vi "ActionVIOnLoad.vi"(8 "error in (no error)":errorcluster, 11 "Device Item Ref in":T1 format="%.0x") -> (0 "error out":errorcluster, 3 "Device Item Ref out":T1 format="%.0x")   [LabVIEW 2015, in "Fuel Injector Analysis Addon System Explorer.lvlib"]
uses:
  Fuel Injector Analysis Addon System Explorer.lvlib
  <vilib>/NI Veristand/Custom Device API/Custom Device Item Ref.ctl
  NationalInstruments.VeriStand.SystemDefinitionAPI
  Shared/Constants.vi
  <vilib>/NI Veristand/Custom Device Tools/Custom Device Utility Library/NI VeriStand - Search for Item by GUID.vi
  <vilib>/NI Veristand/Custom Device Tools/Custom Device Utility Library/NI VeriStand - Search for All Items by GUID.vi
  <vilib>/NI Veristand/Custom Device API/Custom Device API.lvlib
  <vilib>/NI Veristand/Custom Device Tools/Custom Device Utility Library/Custom Device Utility Library.lvlib
  Shared/Fuel Injector Analysis Addon Shared.lvlib
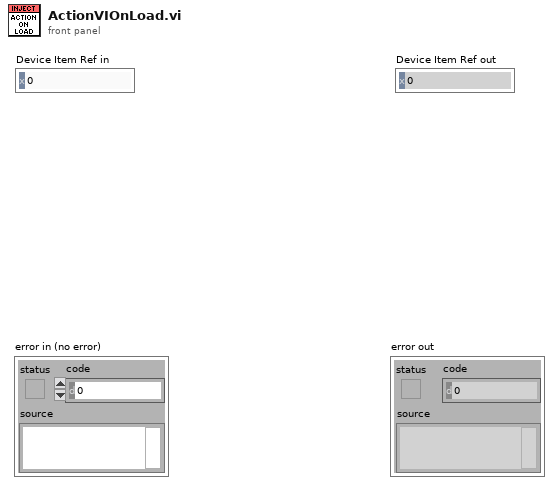
[diagram p1: front panel]
types:
  T1 = typedef "Custom Device API.lvlib/Custom Device Item Ref.ctl" = u64
  T2 = typedef "Fuel Injector Analysis Addon Shared.lvlib/Analysis.Channels.Select.ctl" = cluster{"Pull In Time":bool, "Pull In Max Current":bool, "Pull In Max Voltage":bool, "Pull In Min Voltage":bool, "Pull In Avg Voltage":bool, "Hold Time":bool, "Hold Max Current":bool, "Hold Min Current":bool, "Hold Avg Current":bool, "Hold Max Voltage":bool, "Hold Min Voltage":bool, "Hold Avg Max Voltage":bool, "Hold Avg Min Voltage":bool, "Off Time":bool, "Off Max Current":bool, "Off Min Current":bool, "Off Avg Current":bool, "Off Max Voltage":bool, "Off Min Voltage":bool, "Off Avg Voltage":bool, "Total Voltage Pulses":bool, "Total Stage Time":bool}
  T3 = typedef "Custom Device API.lvlib/Custom Device Item Info.ctl" = cluster{"Name":string, "Is Channel":bool, "GUID":string, "Is Waveform":bool}
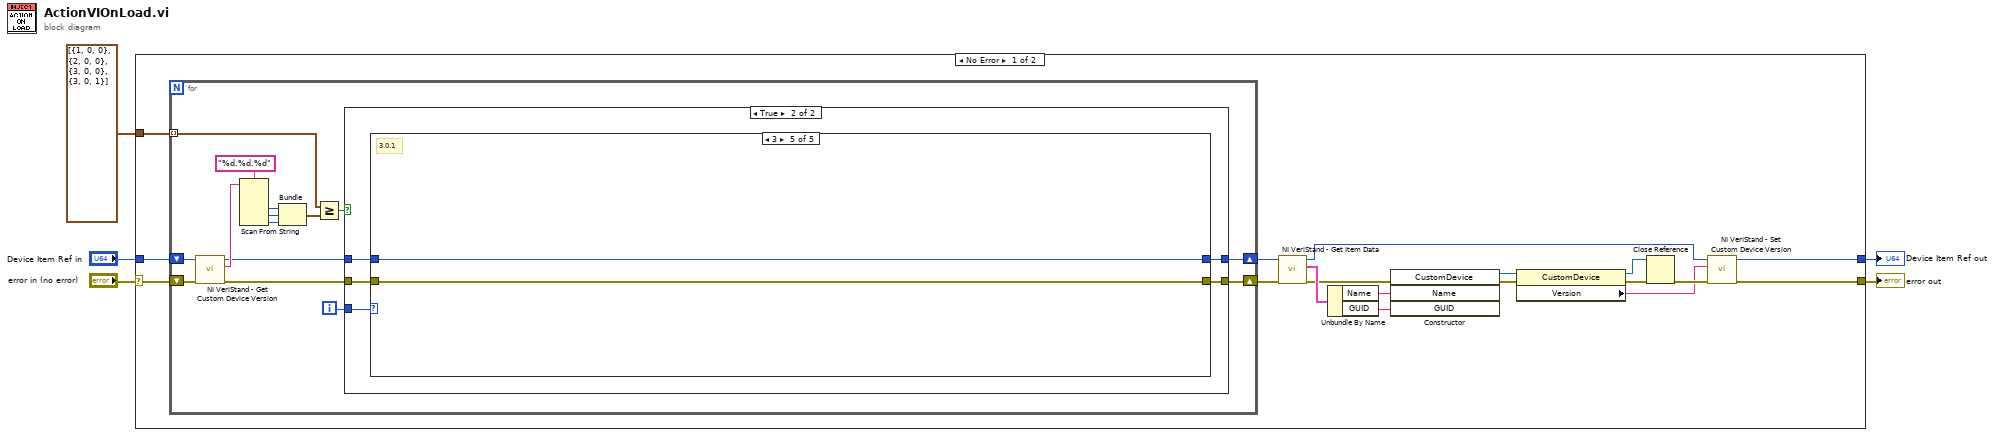
[diagram p0: block diagram]
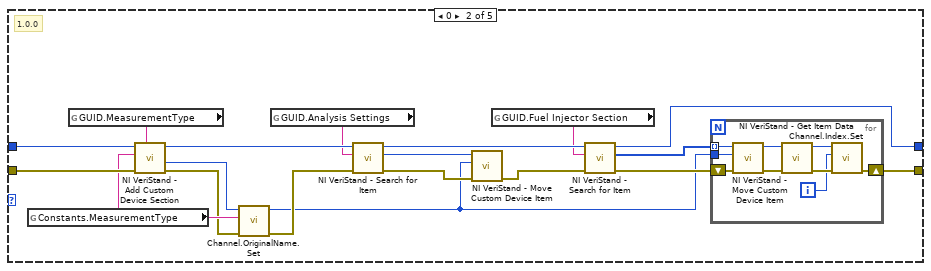
[diagram p4: hidden frame]
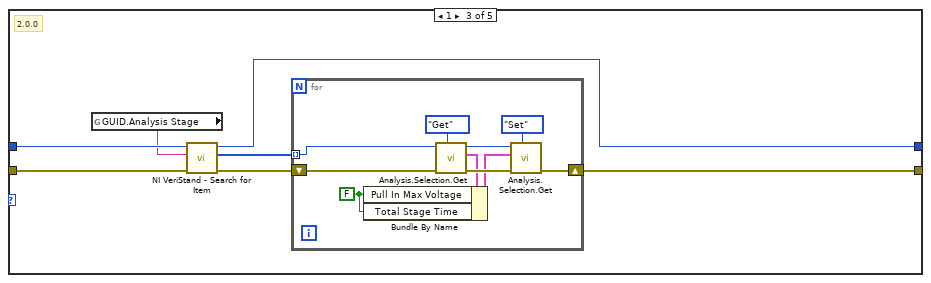
[diagram p5: hidden frame]
diagram:
  n1 = case shown="No Error" "error in (no error)" {
    selector: "error in (no error)" -> [w22 w98]
    tunnel: [w8 w98] -> w2
    tunnel: "Device Item Ref in" -> [w21 w97]
    tunnel: [w6 w97] -> w1
    tunnel: cluster{i32, i32, i32}[] [{1, 0, 0}, {2, 0, 0}, {3, 0, 0}, {3, 0, 1}] -> [w23 _]
    frame No Error {
      n2 = for {
        tunnel: w23 -> [w26] mode=indexing
        shift-right: [w31] -> w9
        shift-left: w22 -> [w36]
        shift-right: [w29] -> w7
        shift-left: w21 -> [w35]
        i -> [w28]
        n3 = call <vilib>:"NI VeriStand - Get Custom Device Version.vi"("error in (no error)"=w36, "Device Ref in"=w35) -> ("error out"=w32:errorcluster, "Value"=w34:string, "Device Ref out"=w30:T1)  [unwired: 7 in]
        n4 = Scan From String(format string="%d.%d.%d", input string=w34) -> (output 1=w37:i32, output 2=w38:i32, output 3=w25:i32)  [unwired: 5 in, 3 out]
        n5 = Bundle(w37, w38, w25) -> (w24:cluster{i32, i32, i32})  [unwired: 1 in]
        n6 = Greater Or Equal?(x=w26, y=w24) -> (x >= y?=w33:bool)
        n7 = case shown="True" w33 {
          tunnel: w32 -> [w40 w45]
          tunnel: [w40 w44] -> w31
          tunnel: w30 -> [w39 w41]
          tunnel: [w39 w42] -> w29
          tunnel: w28 -> [_ w43]
          frame False {
          }
          frame True {
            n8 = case shown="3" w43 {
              tunnel: w45 -> [w47 w66 w82 w94 w96]
              tunnel: [w47 w60 w78 w94 w96] -> w44
              tunnel: [w46 w63 w76 w93 w95] -> w42
              tunnel: w41 -> [w46 w65 w81 w93 w95]
              frame Default {
              }
              frame 0 {
                # "1.0.0"
                n9 = global read "Constants.vi" "Constants.MeasurementType"() -> (w52:string)
                n10 = global read "Constants.vi" "GUID.MeasurementType"() -> (w53:string)
                n11 = call <vilib>:"NI VeriStand - Add Custom Device Section.vi"("GUID (Default Section)"=w53, "error in (no error)"=w66, "Section Name"=w52, "Parent Ref in"=w65) -> ("error out"=w51:errorcluster, "Section Ptr"=w49:T1, "Parent Ref out"=w64:T1)  [unwired: 4 in, 1 out]
                n12 = call "Channel.OriginalName.Set.vi"("error in (no error)"=w51, "Constants.Channel Name"=w52, "Ref"=w49) -> ("error out"=w50:errorcluster, "Ref out"=w48:T1)  [unwired: 7 in]
                n13 = global read "Constants.vi" "GUID.Analysis Settings"() -> (w55:string)
                n14 = call-poly <vilib>:"NI VeriStand - Search for Item.vi"("error in"=w50, "Item GUID"=w55, "Section Ref in"=w64) -> ("error out"=w58:errorcluster, "Item Ref"=w59:T1, "Section Ref out"=w57:T1)  [unwired: 5 in, 1 out]
                n15 = call <vilib>:"NI VeriStand - Move Custom Device Item.vi"("error in (no error)"=w58, "New Parent Ref in"=w48, "Item Ref in"=w59) -> ("error out"=w56:errorcluster)  [unwired: 6 in, 2 out]
                n16 = global read "Constants.vi" "GUID.Fuel Injector Section"() -> (w54:string)
                n17 = call-poly <vilib>:"NI VeriStand - Search for Item.vi"("error in"=w56, "Item GUID"=w54, "Section Ref in"=w57) -> ("error out"=w61:errorcluster, "Item Refs"=w62:T1[], "Section Ref out"=w63:T1)  [unwired: 5 in, 1 out]
                n18 = for {
                  tunnel: w62 -> [w75] mode=indexing
                  shift-right: [w68] -> w60
                  shift-left: w61 -> [w74]
                  tunnel: w48 -> [w73]
                  i -> [w67]
                  n19 = call <vilib>:"NI VeriStand - Move Custom Device Item.vi"("error in (no error)"=w74, "New Parent Ref in"=w73, "Item Ref in"=w75) -> ("error out"=w71:errorcluster, "Item Ref out"=w72:T1)  [unwired: 6 in, 1 out]
                  n20 = call <vilib>:"NI VeriStand - Get Item Data.vi"("error in (no error)"=w71, "Item Ref in"=w72) -> ("error out"=w69:errorcluster, "Item Ref out"=w70:T1)  [unwired: 6 in, 2 out]
                  n21 = call "Channel.Index.Set.vi"("error in (no error)"=w69, "Constants.Index"=w67, "Ref"=w70) -> ("error out"=w68:errorcluster)  [unwired: 7 in, 1 out]
                }
              }
              frame 1 {
                # "2.0.0"
                n22 = global read "Constants.vi" "GUID.Analysis Stage"() -> (w80:string)
                n23 = call-poly <vilib>:"NI VeriStand - Search for Item.vi"("error in"=w82, "Item GUID"=w80, "Section Ref in"=w81) -> ("error out"=w79:errorcluster, "Item Refs"=w77:T1[], "Section Ref out"=w76:T1)  [unwired: 5 in, 1 out]
                n24 = for {
                  shift-right: [w88] -> w78
                  shift-left: w79 -> [w90]
                  tunnel: w77 -> [w83] mode=indexing
                  w84 = FALSE ("Pull In Max Voltage")
                  n25 = call "Analysis.Selection.Get.vi"("Action"=enum8{"Get", "Set"}."Get", "error in (no error)"=w90, "Item Ref in"=w83) -> ("error out"=w89:errorcluster, "Selections"=w86:T2, "Item Ref out"=w87:T1)  [unwired: 6 in]
                  n26 = Bundle By Name(cluster=w86, "Pull In Max Voltage"=w84, "Total Stage Time"=w84) -> (w85:T2)
                  n27 = call "Analysis.Selection.Get.vi"("Action"=enum8{"Get", "Set"}."Set", "error in (no error)"=w89, "Selections"=w85, "Item Ref in"=w87) -> ("error out"=w88:errorcluster)  [unwired: 5 in, 2 out]
                }
              }
              frame 2 {
                # "3.0.0"
              }
              frame 3 {
                # "3.0.1"
              }
            }
          }
        }
      }
      n28 = call <vilib>:"NI VeriStand - Get Item Data.vi"("error in (no error)"=w9, "Item Ref in"=w7) -> ("error out"=w17:errorcluster, "Item Info"=w20:T3, "Item Ref out"=w10:T1)  [unwired: 6 in, 1 out]
      n29 = Unbundle By Name(w20) -> ("Name"=w19:string, "GUID"=w18:string)
      n30 = constructor class="CustomDevice"(error in=w17, "Name"=w19, "GUID"=w18) -> (reference out=w16:refnum<k24>, error out=w15:errorcluster)  [unwired: 2 in, 3 out]
      n31 = property class="CustomDevice"(reference=w16, error in=w15) -> (reference out=w13:refnum<k24>, error out=w14:errorcluster, "Version"=w11:string)
      n32 = Close Reference(reference=w13, error in (no error)=w14) -> (error out=w12:errorcluster)
      n33 = call <vilib>:"NI VeriStand - Set Custom Device Version.vi"("error in (no error)"=w12, "Value"=w11, "Device Ref in"=w10) -> ("error out"=w8:errorcluster, "Device Ref out"=w6:T1)  [unwired: 7 in]
    }
    frame Error {
    }
  }
  "error out" <- w2
  "Device Item Ref out" <- w1
